vi "File to Array.vi"(8 "error in":errorcluster, 11 "file path in":path) -> (0 "error out":errorcluster, 2 "list out":T1[](array[typedef]) {"Creation Date" format="%<%x>T"; "Last Updated" format="%<%x>T"}, 3 "file path out":path)   [LabVIEW 2018]
uses:
  Type Defs/SR Cluster.ctl
  Type Defs/SR Status.ctl
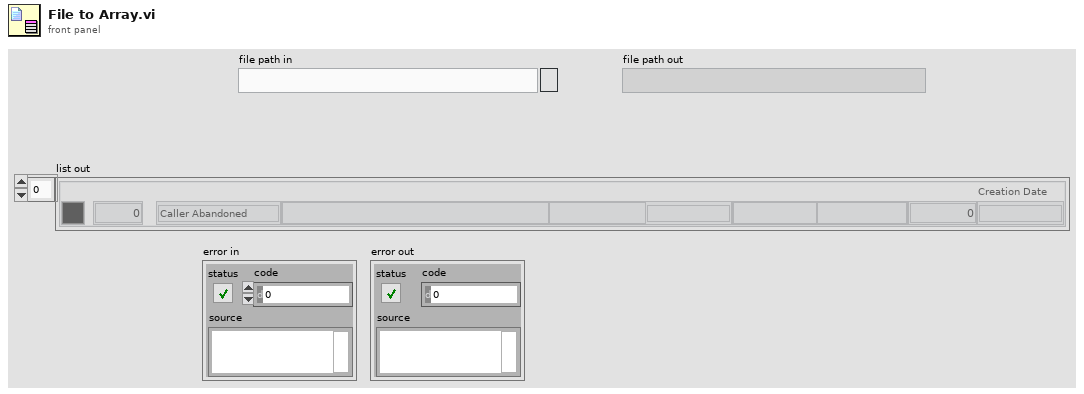
[diagram p1: front panel]
types:
  T1 = typedef "SR Cluster.ctl" = cluster{"Color":u32, "SR Number":i32, "SR Status":T2, "Name":string, "Summary":string, "Last Updated":timestamp, "SR Type":string, "Service Level":string, "Days Open":dbl, "Creation Date":timestamp}
  T2 = typedef "SR Status.ctl" = enum16{"Caller Abandoned", "Created in Error", "Expired", "Forum Resolved AE", "Forum Resolved Customer", "IN WORK", "IN WORK Collab with AES", "IN WORK Collab with PSE", "IN WORK Collab with SE", "IN WORK Customer Added Note", "IN WORK Escalation", "IN WORK Wait on Customer", "Open", "Potentially Resolved", "Presumed Resolved", "RMA Approved for Return", "Resolved", "Passed Off"}
  T3 = enum16{"open", "replace", "create", "open or create", "replace or create", "replace or create with confirmation"}
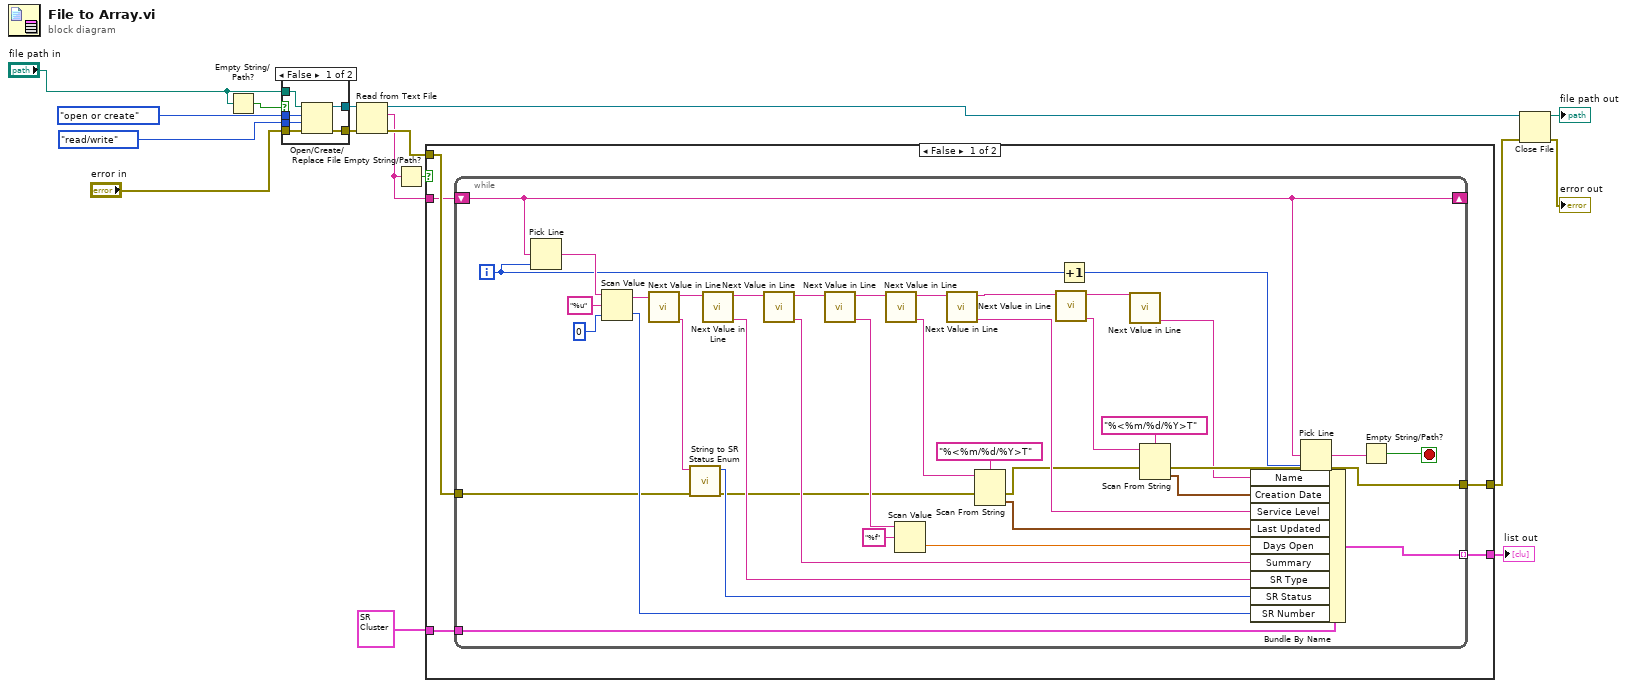
[diagram p0: block diagram]
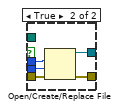
[diagram p2: hidden frame]
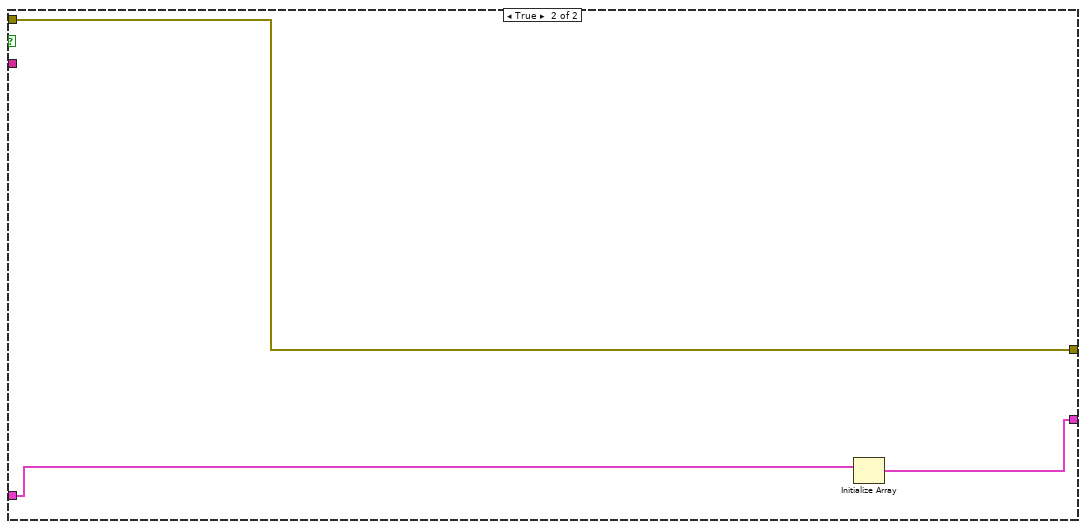
[diagram p3: hidden frame]
diagram:
  n1 = Empty String/Path?(string/path="file path in") -> (empty?=w2:bool)
  n2 = case shown="False" w2 {
    tunnel: enum16{"read/write", "read-only", "write-only"}."read/write" ("access (0:read/write)") -> [w22 w26]
    tunnel: T3."open or create" ("operation (0:open)") -> [w21 w27]
    tunnel: "error in" -> [w20 w25]
    tunnel: [w19 w23] -> w13
    tunnel: [w18 w24] -> w12
    tunnel: "file path in" -> [w17 _]
    frame False {
      n3 = Open/Create/Replace File(file path (use dialog)=w17, error in=w20, operation (0:open)=w21, access (0:read/write)=w22) -> (refnum out=w19:refnum<file>, error out=w18:errorcluster)  [unwired: 2 in, 1 out]
    }
    frame True {
      n4 = Open/Create/Replace File(error in=w25, operation (0:open)=w27, access (0:read/write)=w26) -> (refnum out=w23:refnum<file>, error out=w24:errorcluster)  [unwired: 3 in, 1 out]
    }
  }
  n5 = Read from Text File(file (use dialog)=w13, error in=w12) -> (refnum out=w7:refnum<file>, text=w9:string, error out=w10:errorcluster)  [unwired: 2 in, 1 out]
  n6 = Empty String/Path?(string/path=w9) -> (empty?=w11:bool)
  n7 = case shown="False" w11 {
    tunnel: w10 -> [w31 w71]
    tunnel: w9 -> [w30 _]
    tunnel: T1 {"Color"=0, "SR Number"=0, "SR Status"=enum."Caller Abandoned", "Name"="", "Summary"="", "Last Updated"=timestamp(0 s since 1904-01-01), "SR Type"="", "Service Level"="", "Days Open"=0.0, "Creation Date"=timestamp(0 s since 1904-01-01)} ("SR Cluster") -> [w32 w73]
    tunnel: [w29 w71] -> w6
    tunnel: [w28 w72] -> w5
    frame False {
      n8 = while {
        tunnel: w32 -> [w61]
        tunnel: w31 -> [w42]
        shift-right: [w49] -> _
        shift-left: w30 -> [w49]
        tunnel: [w50] -> w28 mode=indexing
        tunnel: [w35] -> w29
        i -> [w46]
        stop <- w47 stop-if-true
        n9 = Pick Line(multi-line string=w49, line index=w46) -> (output string=w70:string)  [unwired: 1 in]
        n10 = Scan Value(string=w70, format string="%u", default (0 dbl)=0) -> (output string=w67:string, value=w60:i32)
        n11 = call "Next Value in Line.vi"("string in"=w67) -> ("value"=w44:string, "rest of string"=w66:string)  [unwired: 9 in]
        n12 = call "String to SR Status Enum.vi"("error in"=w42, "string in"=w44) -> ("error out"=w41:errorcluster, "SR Status"=w43:T2)  [unwired: 8 in]
        n13 = call "Next Value in Line.vi"("string in"=w66) -> ("value"=w59:string, "rest of string"=w65:string)  [unwired: 9 in]
        n14 = call "Next Value in Line.vi"("string in"=w65) -> ("value"=w58:string, "rest of string"=w64:string)  [unwired: 9 in]
        n15 = call "Next Value in Line.vi"("string in"=w64) -> ("value"=w56:string, "rest of string"=w63:string)  [unwired: 9 in]
        n16 = call "Next Value in Line.vi"("string in"=w63) -> ("value"=w54:string, "rest of string"=w62:string)  [unwired: 9 in]
        n17 = Scan Value(string=w56, format string="%f") -> (value=w57:dbl)  [unwired: 1 in, 1 out]
        n18 = call "Next Value in Line.vi"("string in"=w62) -> ("value"=w51:string, "rest of string"=w40:string)  [unwired: 9 in]
        n19 = Scan From String(format string="%<%m/%d/%Y>T", input string=w54, error in=w41) -> (error out=w36:errorcluster, output 1=w52:timestamp)  [unwired: 2 in, 2 out]
        n20 = call "Next Value in Line.vi"("string in"=w40) -> ("value"=w39:string, "rest of string"=w34:string)  [unwired: 9 in]
        n21 = Increment(x=w46) -> (x+1=w45:i32)
        n22 = call "Next Value in Line.vi"("string in"=w34) -> ("value"=w33:string)  [unwired: 9 in, 1 out]
        n23 = Scan From String(format string="%<%m/%d/%Y>T", input string=w39, error in=w36) -> (error out=w35:errorcluster, output 1=w37:timestamp)  [unwired: 2 in, 2 out]
        n24 = Bundle By Name(cluster=w61, "Name"=w33, "Creation Date"=w37, "Service Level"=w51, "Last Updated"=w52, "Days Open"=w57, "Summary"=w58, "SR Type"=w59, "SR Status"=w43, "SR Number"=w60) -> (w50:T1)
        n25 = Pick Line(multi-line string=w49, line index=w45) -> (output string=w48:string)  [unwired: 1 in]
        n26 = Empty String/Path?(string/path=w48) -> (empty?=w47:bool)
      }
    }
    frame True {
      n27 = Initialize Array(w73) -> (w72:T1[])  [unwired: 1 in]
    }
  }
  "list out" <- w5
  n28 = Close File(refnum=w7, error in=w6) -> (path=→"file path out":path, error out=→"error out":errorcluster)
